vi "RT_Aerodynamic_Moment_due_to_Fins_Misalignment (SubVI).vi"(4 "Sref [m^2]":dbl, 6 "Dref":dbl=1.72 format="%#_13g", 7 "Pdin [Pa]":dbl, 8 "DCM":dbl[][](array[numeric]), 9 "i":i32, 10 "dl [rad] in":dbl, 11 "Data":dbl[][](array[numeric])) -> (3 "MA_f":dbl[](array[numeric]))   [LabVIEW 2017]
uses:
  <vilib>/Analysis/baseanly.llb/Real A x B.vi
  <vilib>/Analysis/Matrix/Numeric/Conversions/Array To Matrix - RA2.vi
  <vilib>/Analysis/Matrix/Numeric/Conversions/Array To Matrix - RA.vi
  <vilib>/Analysis/Matrix/Numeric/Conversions/Matrix To Array - RM.vi
  <vilib>/Analysis/NI_AALBase.lvlib
  <vilib>/Analysis/Matrix/NI_Matrix.lvlib
panel:
  out "ma_f":dbl
  out "Cld":dbl
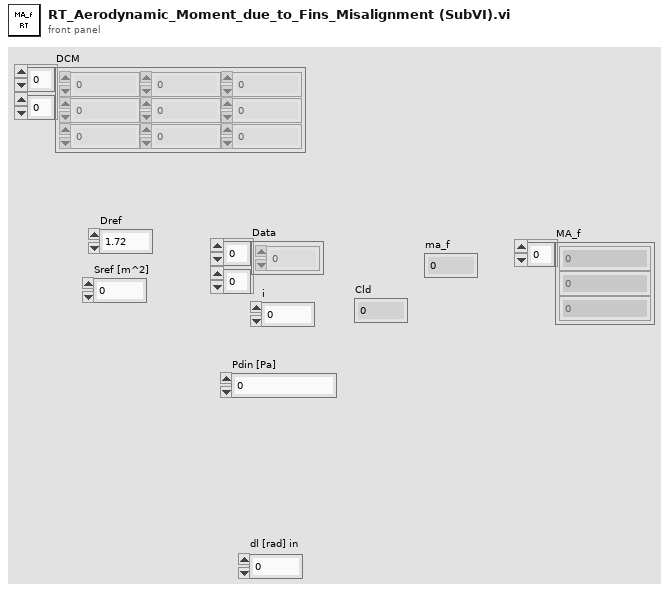
[diagram p1: front panel]
types:
  T1 = typedef "NI_Matrix.lvlib/RealMatrix.ctl" = dbl[][]
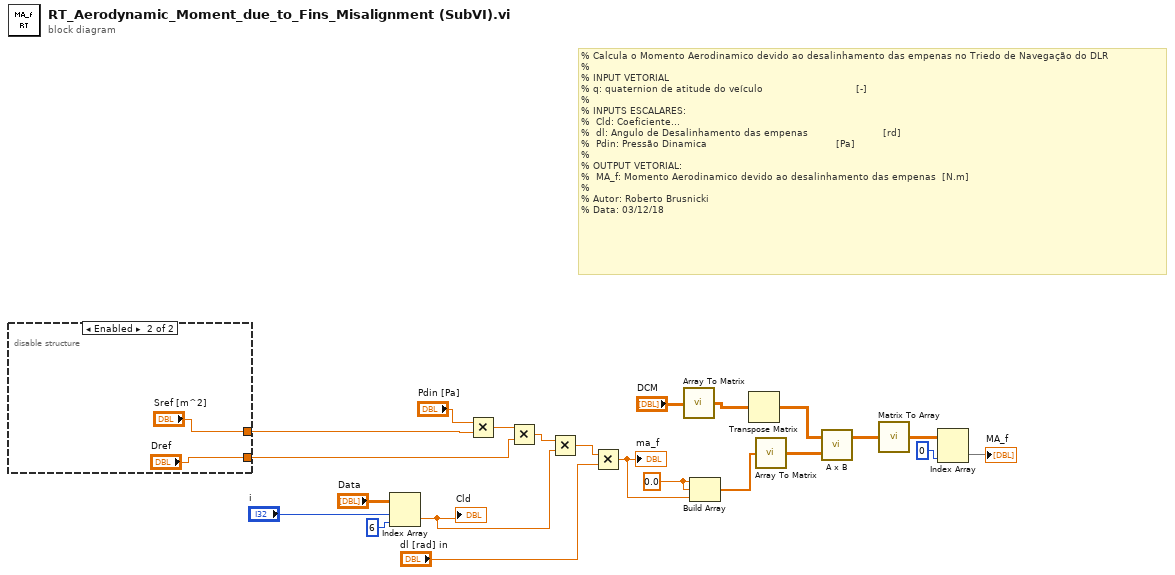
[diagram p0: block diagram]
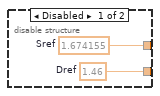
[diagram p2: hidden frame]
diagram:
  w10 = 0.0 ("element")
  # "% Calcula o Momento Aerodinamico devido ao desalinhamento das empenas no Triedo de Navegação do DLR\n%\n% INPUT VETORIAL\n% q: quaternion de atitude do veículo                               [-]\n%\n% INPUTS ESCALARES:\n%  Cld: Coeficiente...\n%  dl: Angulo de Desalinhamento das empenas                         [rd]\n%  Pdin: Pressão Dinamica                                           [Pa]\n%\n% OUTPUT VETORIAL:\n%  MA_f: Momento Aerodinamico devido ao desalinhamento das empenas  [N.m]\n%\n% Autor: Roberto Brusnicki\n% Data: 03/12/18"
  n1 = disable-structure shown="Enabled" {
    disable-tunnel: [w24 "Sref [m^2]"] -> w19
    disable-tunnel: [w23 "Dref"] -> w16
    frame Disabled {
      w24 = 1.674155  # Sref
      w23 = 1.46  # Dref
    }
    frame Enabled {
    }
  }
  n2 = Index Array(array="Data", index (row)="i", index (col)=6 ("disabled index (col)")) -> (element=w14:dbl)
  "Cld" <- w14
  n3 = Multiply(x="Pdin [Pa]", y=w19) -> (x*y=w17:dbl)
  n4 = Multiply(x=w17, y=w16) -> (x*y=w15:dbl)
  n5 = Multiply(x=w15, y=w14) -> (x*y=w13:dbl)
  n6 = Multiply(x=w13, y="dl [rad] in") -> (x*y=w11:dbl)
  "ma_f" <- w11
  n7 = call-poly <vilib>:"Array To Matrix.vi"("Real 2D Array"="DCM") -> ("Real Matrix"=w3:T1)
  n8 = Build Array(w10, w10, w11) -> (w4:dbl[])
  n9 = Transpose Matrix(1:w3) -> (0:w2:T1)
  n10 = call-poly <vilib>:"Array To Matrix.vi"("Real 1D Array"=w4) -> ("Real Matrix (Column Vector)"=w9:T1)
  n11 = call-poly <vilib>:"A x B.vi"("B"=w9, "A"=w2) -> ("A x B"=w7:T1)  [unwired: 1 out]
  n12 = call-poly <vilib>:"Matrix To Array.vi"("Real Matrix"=w7) -> ("Real 2D Array"=w8:dbl[][])
  n13 = Index Array(array=w8, index (col)=0 ("index (row)")) -> (element=→"MA_f":dbl[])  [unwired: 1 in]
